vi "TagContainer-Flush.vi"(8 "error in (no error)":errorcluster, 11 "TagContainer":T1) -> (0 "error out":errorcluster, 3 "TagContainer(dup)":T1)   [LabVIEW 2017, in "TagContainer.lvlib"]
doc: "Clear all current Tags in Container."
uses:
  TagContainer.lvlib
  Typedef/TagContainer.ctl
panel:
  # "Connector Pane"
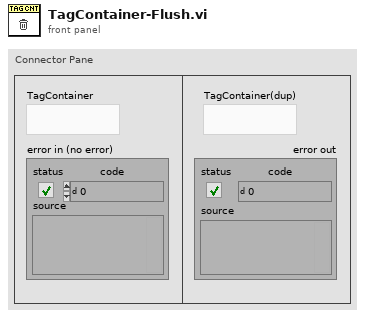
[diagram p1: front panel]
types:
  T1 = typedef "TagContainer.lvlib/TagContainer.ctl" = refnum<k1>
  T2 = typedef "TagContainer.lvlib/tagcontainer-data.ctl" = cluster{"tag-map":variant, "timestamp-map":variant, "namecacher-map":variant, "DataTypeCacher-map":variant, "Tag Adding Lock?":bool, "Global Change Timestamp":timestamp}
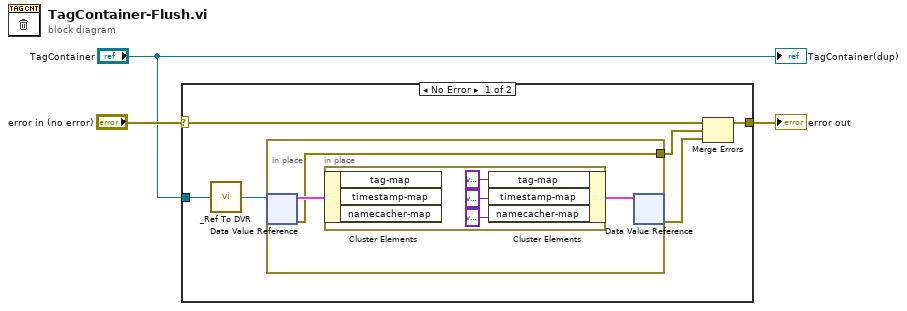
[diagram p0: block diagram]
diagram:
  n1 = case shown="No Error" "error in (no error)" {
    selector: "error in (no error)" -> [w8 w16]
    tunnel: [w9 w16] -> w2
    tunnel: "TagContainer" -> [w7 _]
    frame No Error {
      n2 = call "_Ref To DVR.vi"("TagContainer"=w7) -> ("DVR"=w6:refnum<data-value>)
      n3 = in-place "In Place Element Structure" {
        in-place-border: [w10] -> w5
        n4 = in-place-dvr #1(w6) -> (w12:T2, w10:errorcluster)
        n5 = in-place {
          n6 = in-place-cluster #2(w12) -> ()  [unwired: 3 out]
          n7 = in-place-cluster #2("tag-map"=variant, "timestamp-map"=variant, "namecacher-map"=variant) -> (w11:T2)
        }
        n8 = in-place-dvr #1(w11) -> (w4:errorcluster)  [unwired: 1 out]
      }
      n9 = Merge Errors(w8, w5, w4) -> (w9:errorcluster)
    }
    frame Error {
    }
  }
  "error out" <- w2
  "TagContainer(dup)" <- "TagContainer"
